vi "clearState.vi"(8 "error in (no error)":errorcluster, 11 "ElectrometerController in":refnum<class "ElectrometerController.lvclass">) -> (0 "error out":errorcluster, 3 "ElectrometerController out":refnum<class "ElectrometerController.lvclass">)   [LabVIEW 2016, in "ElectrometerController.lvclass"]
uses:
  ElectrometerController.lvclass
  Electrometer/State/State.lvclass
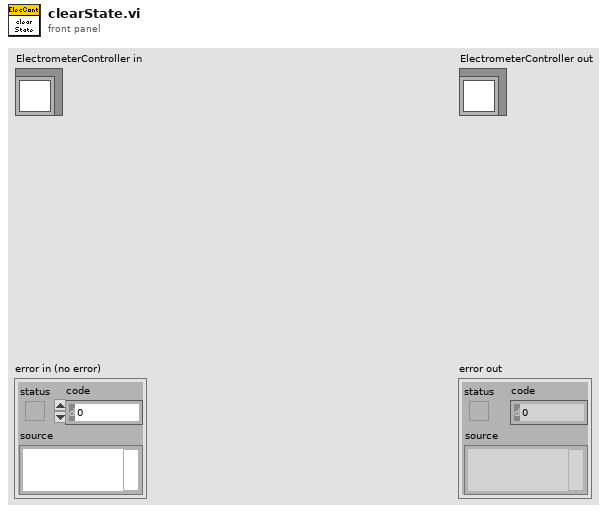
[diagram p1: front panel]
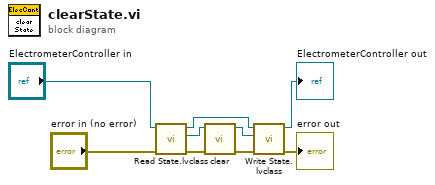
[diagram p0: block diagram]
diagram:
  n1 = call-dynamic "Read State.lvclass.vi"("error in (no error)"="error in (no error)", "ElectrometerController in"="ElectrometerController in") -> ("error out"=w6:errorcluster, "State.lvclass"=w7:refnum<class "State.lvclass">, "ElectrometerController out"=w1:refnum<class "ElectrometerController.lvclass">)  [unwired: 7 in]
  n2 = call-dynamic "clear.vi"("error in (no error)"=w6, "State in"=w7) -> ("error out"=w5:errorcluster, "State out"=w4:refnum<class "State.lvclass">)  [unwired: 8 in]
  n3 = call-dynamic "Write State.lvclass.vi"("error in (no error)"=w5, "State.lvclass"=w4, "ElectrometerController in"=w1) -> ("error out"=→"error out":errorcluster, "ElectrometerController out"=→"ElectrometerController out":refnum<class "ElectrometerController.lvclass">)  [unwired: 7 in]
